vi "lvdt keyence tester.vi"() -> ()   [LabVIEW 2018]
panel:
  out "Waveform Chart":dbl[][](graph)=[[0.49, 0.49, 0.0]]
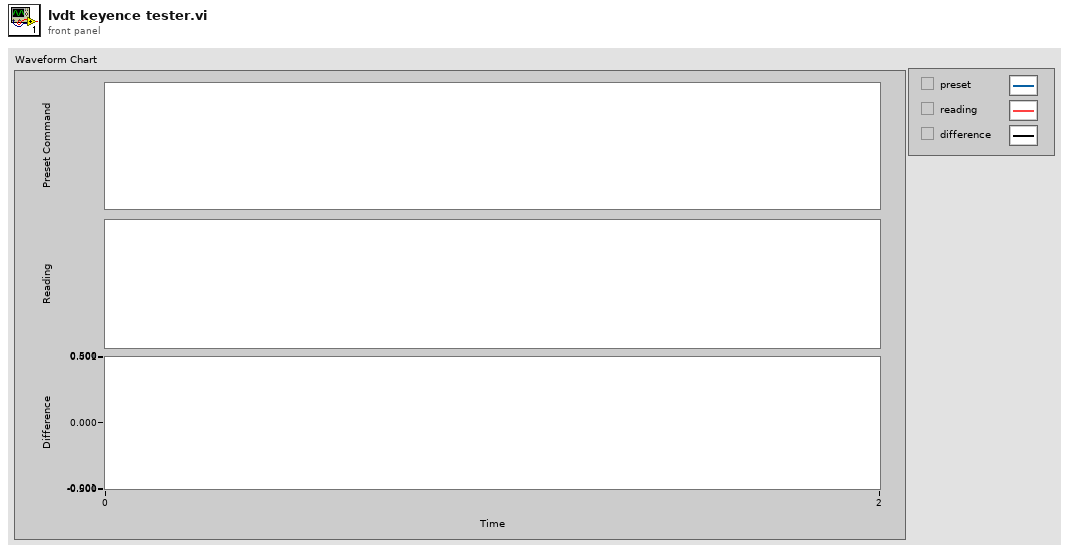
[diagram p1: front panel]
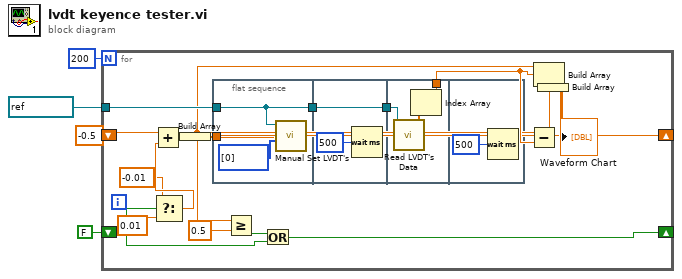
[diagram p0: block diagram]
diagram:
  n1 = for {
    N: 200 -> [_]
    tunnel: refnum<visa-resource-name> "COM9" ("LVDT's 1") -> [w18]
    shift-right: [w10] -> _
    shift-left: FALSE -> [w8]
    shift-right: [w9] -> _
    shift-left: -0.5 -> [w21]
    n2 = Select(t=-0.01, s=w8, f=0.01) -> (s? t:f=w6:dbl)
    n3 = Add(x=w21, y=w6) -> (x+y=w9:dbl)
    n4 = Build Array(w9) -> (w17:dbl[])
    n5 = flat-sequence {
      tunnel: [w24] -> w19
      tunnel: w18 -> [w24]
      tunnel: w17 -> [w23]
      tunnel: [w26] -> w20
      tunnel: w19 -> [w26]
      tunnel: w20 -> [w29]
      tunnel: [w27] -> w14
      frame #0 {
        n6 = call "Manual Set LVDT's.vi"("LVDT Numbers"=i32[] [0], "Data"=w23, "LVDT's 1"=w24) -> ()  [unwired: 7 in, 2 out]
      }
      frame #1 {
        n7 = Wait (ms)(milliseconds to wait=u32 500) -> ()  [unwired: 1 out]
      }
      frame #2 {
        n8 = call "Read LVDT's Data.vi"("LVDT's Com Port"=w29) -> ("Array"=w28:sgl[])  [unwired: 9 in, 1 out]
        n9 = Index Array(array=w28) -> (element=w27:sgl)  [unwired: 1 in]
      }
      frame #3 {
        n10 = Wait (ms)(milliseconds to wait=u32 500) -> ()  [unwired: 1 out]
      }
    }
    n11 = Greater Or Equal?(x=w9, y=0.5) -> (x >= y?=w11:bool)
    n12 = Or(x=w11, y=w8) -> (x .or. y?=w10:bool)
    n13 = Subtract(x=w9, y=w14) -> (x-y=w13:dbl)
    n14 = Build Array(w9, w14, w13) -> (w16:dbl[])
    n15 = Build Array(w16) -> (→"Waveform Chart":dbl[][])
  }
